vi "output_config.vi"(8 "Nazat":bool, 9 "Tam":bool, 10 "We w tê":bool, 11 "W tê":bool) -> (2 "Values":bool[](array[boolean]), 3 "DO Channels":u8[](array[numeric]))   [LabVIEW 2014]
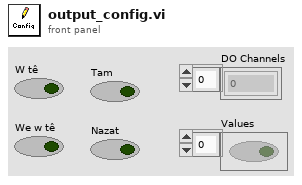
[diagram p1: front panel]
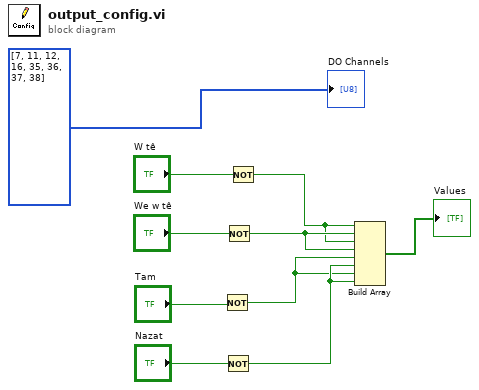
[diagram p0: block diagram]
diagram:
  n1 = Not(x="Tam") -> (.not. x?=w1:bool)
  n2 = Not(x="Nazat") -> (.not. x?=w2:bool)
  n3 = Not(x="We w tê") -> (.not. x?=w10:bool)
  n4 = Not(x="W tê") -> (.not. x?=w9:bool)
  n5 = Build Array(w9, w10, w9, w10, w1, w2, w1, w2) -> (→"Values":bool[])
  "DO Channels" <- u8[] [7, 11, 12, 16, 35, 36, 37, 38] ("DO Channels")
